vi "Configure Control AI Range(RTD).vi"(0 "VISA resource name":refnum<visa-resource-name>, 1 "Unit No. (0)":i32 min=0 max=6, 3 "Type and Span":T1={"RTD Type (0 : Pt100)"=0, "Enable Span (False)"=FALSE, "Lower Span (-200.0)"=-200.0, "Upper Span (850.0)"=850.0, "Bias (0)"=0.0} {"Bias (0)" format="%_6g"; "Upper Span (850.0)" min=-99999.0 max=99999.0 step=0.1 format="%.2f"; "Lower Span (-200.0)" min=-99999.0 max=99999.0 step=0.1 format="%.2f"; "RTD Type (0 : Pt100)" items=["Pt100", "Pt100-H", "JPt100", "JPt100-H", "Cu10GE", "Cu10LN", "Cu10WEED", "Cu10BAILEY", "Cu10a392", "Cu10a393", "Cu25", "Cu53", "Cu100", "J263B", "Ni100SAMA", "Ni100DIN", "Ni120", "Pt25", "Pt50", "Pt200WEED", "Cu10G", "Cu50G", "Cu100G", "Pt46G", "Pt100G"]}, 4 "Module No.(0)":i32 min=0 max=9, 5 "AI No.(1)":i32=1 min=1 max=2, 7 "error in (no error)":errorcluster) -> (20 "VISA resource name out":refnum<visa-resource-name>, 21 "AI No.":i32, 24 "Unit No.":i32, 25 "Module No.":i32, 27 "error out":errorcluster)   [LabVIEW 2020, in "Yokogawa GX Series.lvlib"]
doc: "Set RTD range of AI channel in PID module.\n\nCommand: SCtrlRangeAI"
uses:
  <instrlib>/Yokogawa GX Series/Yokogawa GX Series.lvlib
  <instrlib>/Yokogawa GX Series/Private/RTD Range.vi
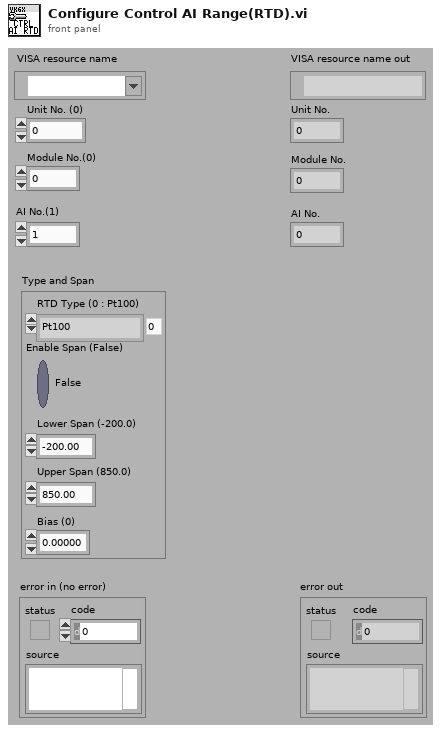
[diagram p1: front panel]
types:
  T1 = cluster{"RTD Type (0 : Pt100)":i32, "Enable Span (False)":bool, "Lower Span (-200.0)":dbl, "Upper Span (850.0)":dbl, "Bias (0)":dbl}
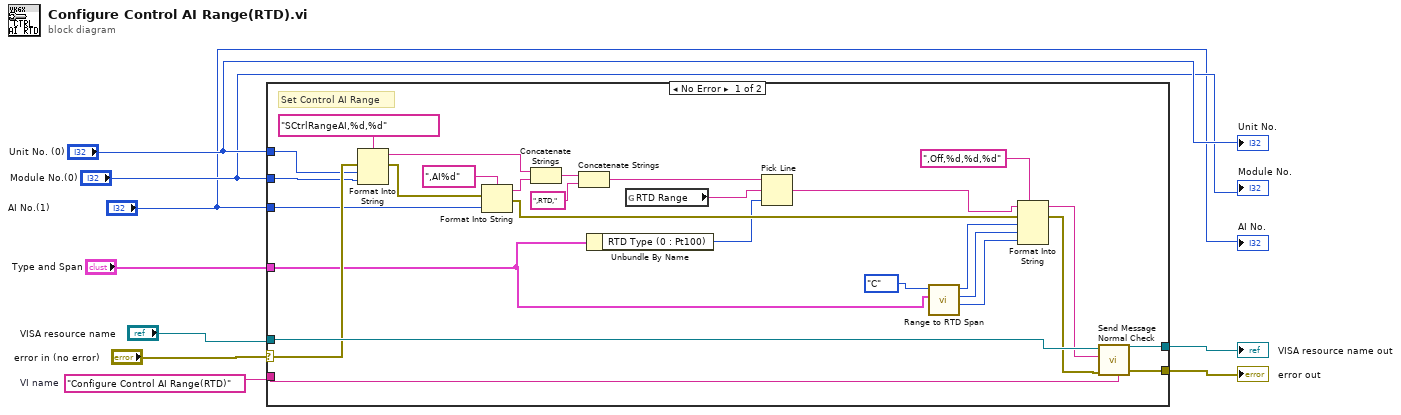
[diagram p0: block diagram]
diagram:
  w5 = "Configure Control AI Range(RTD)"  # VI name
  n1 = case shown="No Error" "error in (no error)" {
    selector: "error in (no error)" -> [w33 w38]
    tunnel: [w37 w39] -> w9
    tunnel: [w36 w38] -> w8
    tunnel: "VISA resource name" -> [w35 w39]
    tunnel: w5 -> [w32 _]
    tunnel: "Unit No. (0)" -> [w31 _]
    tunnel: "Module No.(0)" -> [w30 _]
    tunnel: "AI No.(1)" -> [w28 _]
    tunnel: "Type and Span" -> [w14 _]
    frame No Error {
      # "Set Control AI Range"
      n2 = Format Into String(format string="SCtrlRangeAI,%d,%d", error in=w33, w31, w30) -> (resulting string=w26:string, error out=w27:errorcluster)  [unwired: 1 in]
      n3 = Format Into String(format string=",AI%d", error in=w27, w28) -> (resulting string=w25:string, error out=w20:errorcluster)  [unwired: 1 in]
      n4 = Concatenate Strings(w26, w25) -> (w21:string)
      n5 = Concatenate Strings(w21, ",RTD,") -> (w23:string)
      n6 = Unbundle By Name(w14) -> ("RTD Type (0 : Pt100)"=w10:i32)
      n7 = global read "RTD Range.vi" "RTD Range"() -> (w16:string)
      n8 = Pick Line(string ("")=w23, multi-line string=w16, line index=w10) -> (output string=w19:string)
      n9 = call <instrlib>:"Range to RTD Span.vi"("Type and Span"=w14, "Temp. unit (0: C)"=enum16{"C", "F"}."C") -> ("Bias"=w11:i32, "Upper span"=w12:i32, "Lower Span"=w13:i32)  [unwired: 7 in]
      n10 = Format Into String(format string=",Off,%d,%d,%d", initial string=w19, error in=w20, w13, w12, w11) -> (resulting string=w17:string, error out=w18:errorcluster)
      n11 = call <instrlib>:"Send Message Normal Check.vi"("Source (\"\")"=w32, "error in (no error)"=w18, "Send Message (\"\")"=w17, "VISA resource name"=w35) -> ("error out"=w36:errorcluster, "VISA resource name out"=w37:refnum<visa-resource-name>)  [unwired: 2 in, 4 out]
    }
    frame Error {
    }
  }
  "error out" <- w8
  "VISA resource name out" <- w9
  "Unit No." <- "Unit No. (0)"
  "Module No." <- "Module No.(0)"
  "AI No." <- "AI No.(1)"
